vi "testCustomAssertionFailureMessage.vi"() -> ()   [LabVIEW 2017, in "Assertion.Tests.lvlib" / "ErrorMessageContainsString.lvlib"]
uses:
  ErrorMessageContainsString.lvlib
  217b4f57-2f31-42df-b5ae-10c04b4f12b7.vi
  Constraint/IsEqual/Create.vi
  Constraint/IsEqual/IsEqual.lvclass
  Assertion/Assertion.lvlib
  Assertion.Tests.lvlib
panel:
  out "error out":errorcluster
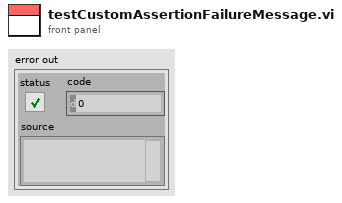
[diagram p1: front panel]
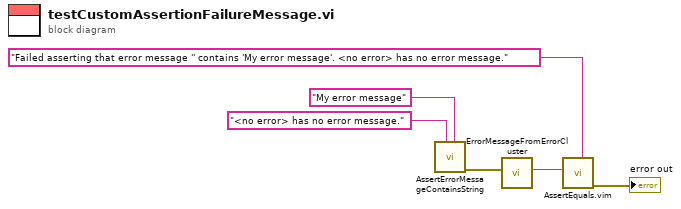
[diagram p0: block diagram]
diagram:
  n1 = call "AssertErrorMessageContainsString.vi"("Expected"="My error message", "Message (\"\")"="<no error> has no error message." ("Message (\"\")")) -> ("error out"=w2:errorcluster)  [unwired: 9 in]
  n2 = call "ErrorMessageFromErrorCluster.vi"("Error"=w2) -> ("Error Message"=w1:string)  [unwired: 10 in]
  n3 = call "AssertEquals.vim"("Expected"="Failed asserting that error message '' contains 'My error message'. <no error> has no error message." ("Needle"), "Actual"=w1) -> ("error out"=→"error out":errorcluster)  [unwired: 9 in]
